vi "DQ subVI.vi"(9 "window (h)":i32, 11 "XY-data":cluster{"X-array":dbl[], "Y-array":dbl[]}) -> (3 "XY-data":cluster{"X-array":dbl[], "Y-array":dbl[]})   [LabVIEW 2019, in "xy_utilities.lvlib"]
doc: "Difference Quotient subVI"
uses:
  xy_utilities.lvlib
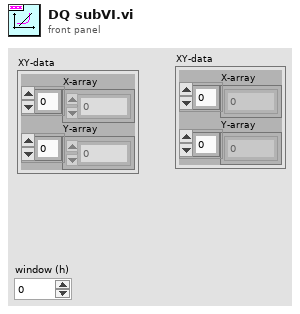
[diagram p1: front panel]
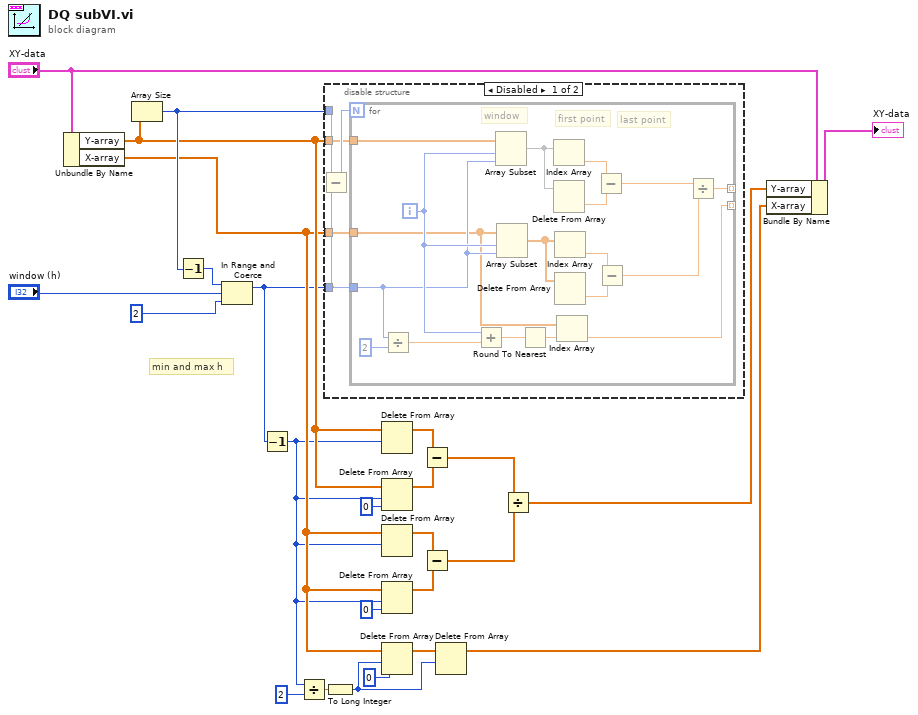
[diagram p0: block diagram]
diagram:
  # "min and max h"
  n1 = Unbundle By Name("XY-data") -> ("Y-array"=w10:dbl[], "X-array"=w9:dbl[])
  n2 = Array Size(array=w10) -> (size(s)=w21:i32)
  n3 = Decrement(x=w21) -> (x-1=w22:i32)
  n4 = In Range and Coerce(upper limit=w22, x="window (h)", lower limit=2) -> (coerced(x)=w7:i32)  [unwired: 1 out]
  n5 = Decrement(x=w7) -> (x-1=w6:i32)
  n6 = Divide(x=w6, y=2) -> (x/y=w4:dbl)
  n7 = disable-structure shown="Disabled" {
    disable-tunnel: w21 -> [w30 _]
    disable-tunnel: w10 -> [w28 _]
    disable-tunnel: w9 -> [w27 _]
    disable-tunnel: w7 -> [w26 _]
    frame Disabled {
      n8 = Subtract(x=w30, y=w26) -> (x-y=w29:i32)
      n9 = for {
        N: w29 -> [_]
        tunnel: w28 -> [w48]
        tunnel: w27 -> [w31]
        tunnel: w26 -> [w32]
        tunnel: [w41] -> _ mode=indexing
        tunnel: [w34] -> _ mode=indexing
        i -> [w38]
        # "last point"
        # "first point"
        # "window"
        n10 = Divide(x=w32, y=2) -> (x/y=w36:dbl)
        n11 = Add(x=w38, y=w36) -> (x+y=w35:dbl)
        n12 = Array Subset(array=w48, index=w38, length=w32) -> (w47:dbl[])
        n13 = Array Subset(array=w31, index=w38, length=w32) -> (w42:dbl[])
        n14 = Round To Nearest(number=w35) -> (nearest integer value=w33:dbl)
        n15 = Index Array(array=w47) -> (element=w46:dbl)  [unwired: 1 in]
        n16 = Delete From Array(array=w47) -> (deleted portion=w45:dbl)  [unwired: 2 in, 1 out]
        n17 = Index Array(array=w42) -> (element=w43:dbl)  [unwired: 1 in]
        n18 = Delete From Array(array=w42) -> (deleted portion=w44:dbl)  [unwired: 2 in, 1 out]
        n19 = Index Array(array=w31, index=w33) -> (element=w34:dbl)
        n20 = Subtract(x=w46, y=w45) -> (x-y=w40:dbl)
        n21 = Subtract(x=w43, y=w44) -> (x-y=w39:dbl)
        n22 = Divide(x=w40, y=w39) -> (x/y=w41:dbl)
      }
    }
    frame Enabled {
    }
  }
  n23 = To Long Integer(number=w4) -> (32bit integer=w2:i32)
  n24 = Delete From Array(array=w10, length=w6) -> (array with subset deleted=w15:dbl[])  [unwired: 1 in, 1 out]
  n25 = Delete From Array(array=w10, length=w6, index=0) -> (array with subset deleted=w16:dbl[])  [unwired: 1 out]
  n26 = Delete From Array(array=w9, length=w6) -> (array with subset deleted=w18:dbl[])  [unwired: 1 in, 1 out]
  n27 = Delete From Array(array=w9, length=w6, index=0) -> (array with subset deleted=w17:dbl[])  [unwired: 1 out]
  n28 = Delete From Array(array=w9, length=w2, index=0) -> (array with subset deleted=w5:dbl[])  [unwired: 1 out]
  n29 = Subtract(x=w15, y=w16) -> (x-y=w13:dbl[])
  n30 = Subtract(x=w18, y=w17) -> (x-y=w12:dbl[])
  n31 = Delete From Array(array=w5, length=w2) -> (array with subset deleted=w1:dbl[])  [unwired: 1 in, 1 out]
  n32 = Divide(x=w13, y=w12) -> (x/y=w11:dbl[])
  n33 = Bundle By Name(cluster="XY-data", "Y-array"=w11, "X-array"=w1) -> (→"XY-data":cluster{"X-array":dbl[], "Y-array":dbl[]})
